vi "CAN路测试.vi"(5 "滤波方式":u8(ring) items=["Dual Filter", "Single Filter"], 6 "E-U_baud":u32(ring)=393223 items=["0x060003--1000Kbps"=393219, "0x060004--800Kbps"=393220, "0x060007--500Kbps"=393223, "0x1C0008--250Kbps"=1835016, "0x1C0011--125Kbps"=1835025, "0x160023--100Kbps"=1441827, "0x1C002C--50Kbps"=1835052, "0x1600B3--20Kbps"=1441971, "0x1C00E0--10Kbps"=1835232, "0x1C01C1--5Kbps"=1835457], 7 "工作方式":u8(ring) items=["Normal", "Listen Only"], 8 "波特率":T1(ring)=enum."500Kbps", 9 "CAN端口":u16(ring) items=["0", "1"], 10 "设备索引号":u16(ring) items=["0", "1", "2", "3", "4", "5", "6", "7", "8", "9", "10", "11", "12", "13", "14", "15", ""], 11 "CAN卡类型":u32(ring)=4 items=["PCI5121"=1, "PCI9810"=2, "USBCAN1"=3, "USBCAN2"=4, "PCI9820"=5, "PCI5110"=7, "CANLite(mini)"=8, "ISA9620"=9, "ISA5420"=10, "PC104CAN"=11, "DNP9810"=13, "PCI9840B"=14, "PC104C2"=15, "PCI9820I"=16, "pec9920"=18, "USBCAN_E_U"=20, "USBCAN_2E_U"=21]) -> ()   [LabVIEW 2013]
uses:
  data/kerneldlls/usbcan.dll
panel:
  in  "数值 4":i32
  in  "数值 3":i32
  out "错误输出":errorcluster
  in  "数值 2":i32
  in  "数值":i32
  in  "退出":bool
  out "整车CAN测试结果":bool
  out "充电CAN测试结果":bool
  out "结果":i32(listbox)=-1
  in  "充电CAN测试":bool
  in  "整车CAN测试":bool
  out "状态":string
  in  "启动CAN 2":bool caption="启动CAN"
  out "状态 2":bool
  out "CAN初始化成功":bool
  in  "启动CAN":bool
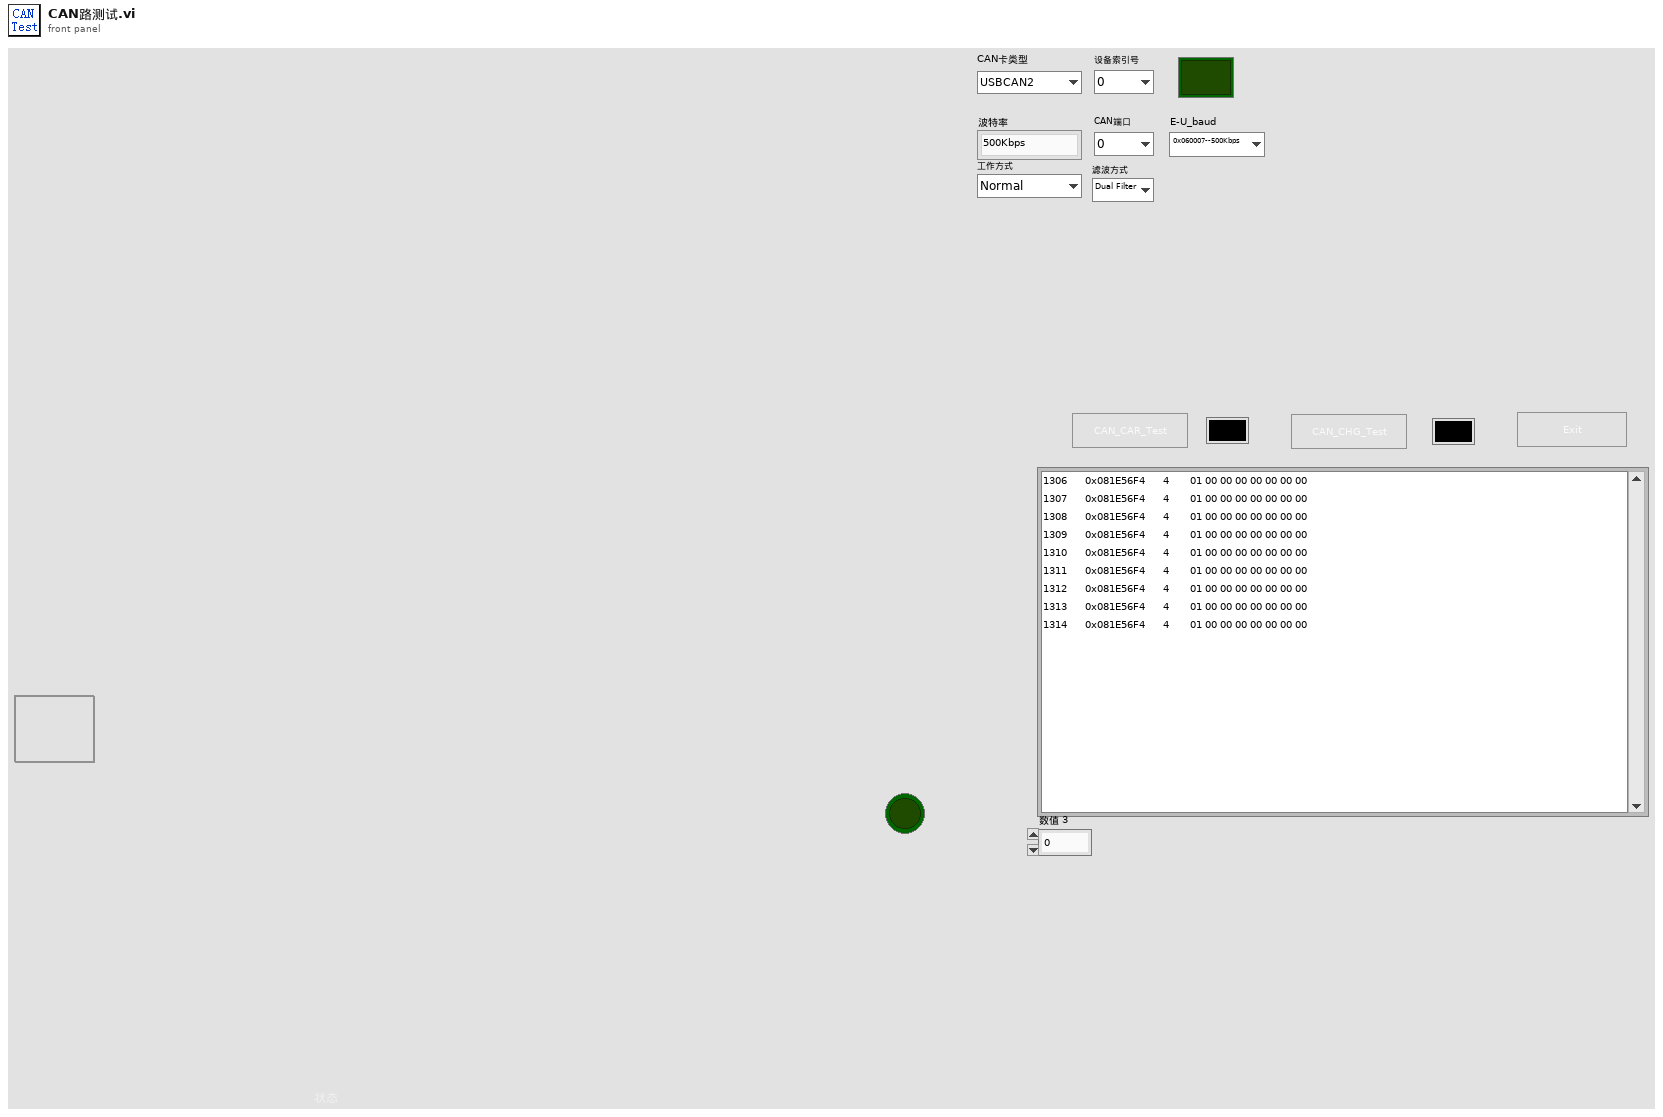
[diagram p1: front panel]
types:
  T1 = enum16{"5Kbps", "10Kbps", "20Kbps", "40Kbps", "50Kbps", "80Kbps", "100Kbps", "125Kbps", "200Kbps", "250Kbps", "400Kbps", "500Kbps", "666Kbps", "800Kbps", "1000Kbps"}
  T2 = cluster{"打开CAN":bool, "初始化CAN":bool, "开始CAN":bool, "重启":bool, "关闭CAN":bool}
  T3 = enum32{"Invalid", "Standard", "Closed", "Hidden", "Minimized", "Maximized"}
  T4 = cluster{"ID":u32, "TimeStamp":u32, "TimeFlag":u8, "SendType":u8, "RemoteFlag":u8, "ExternFlag":u8, "DataLen":u8, u8, u8, u8, u8, u8, u8, u8, u8, u8, u8, u8}[]
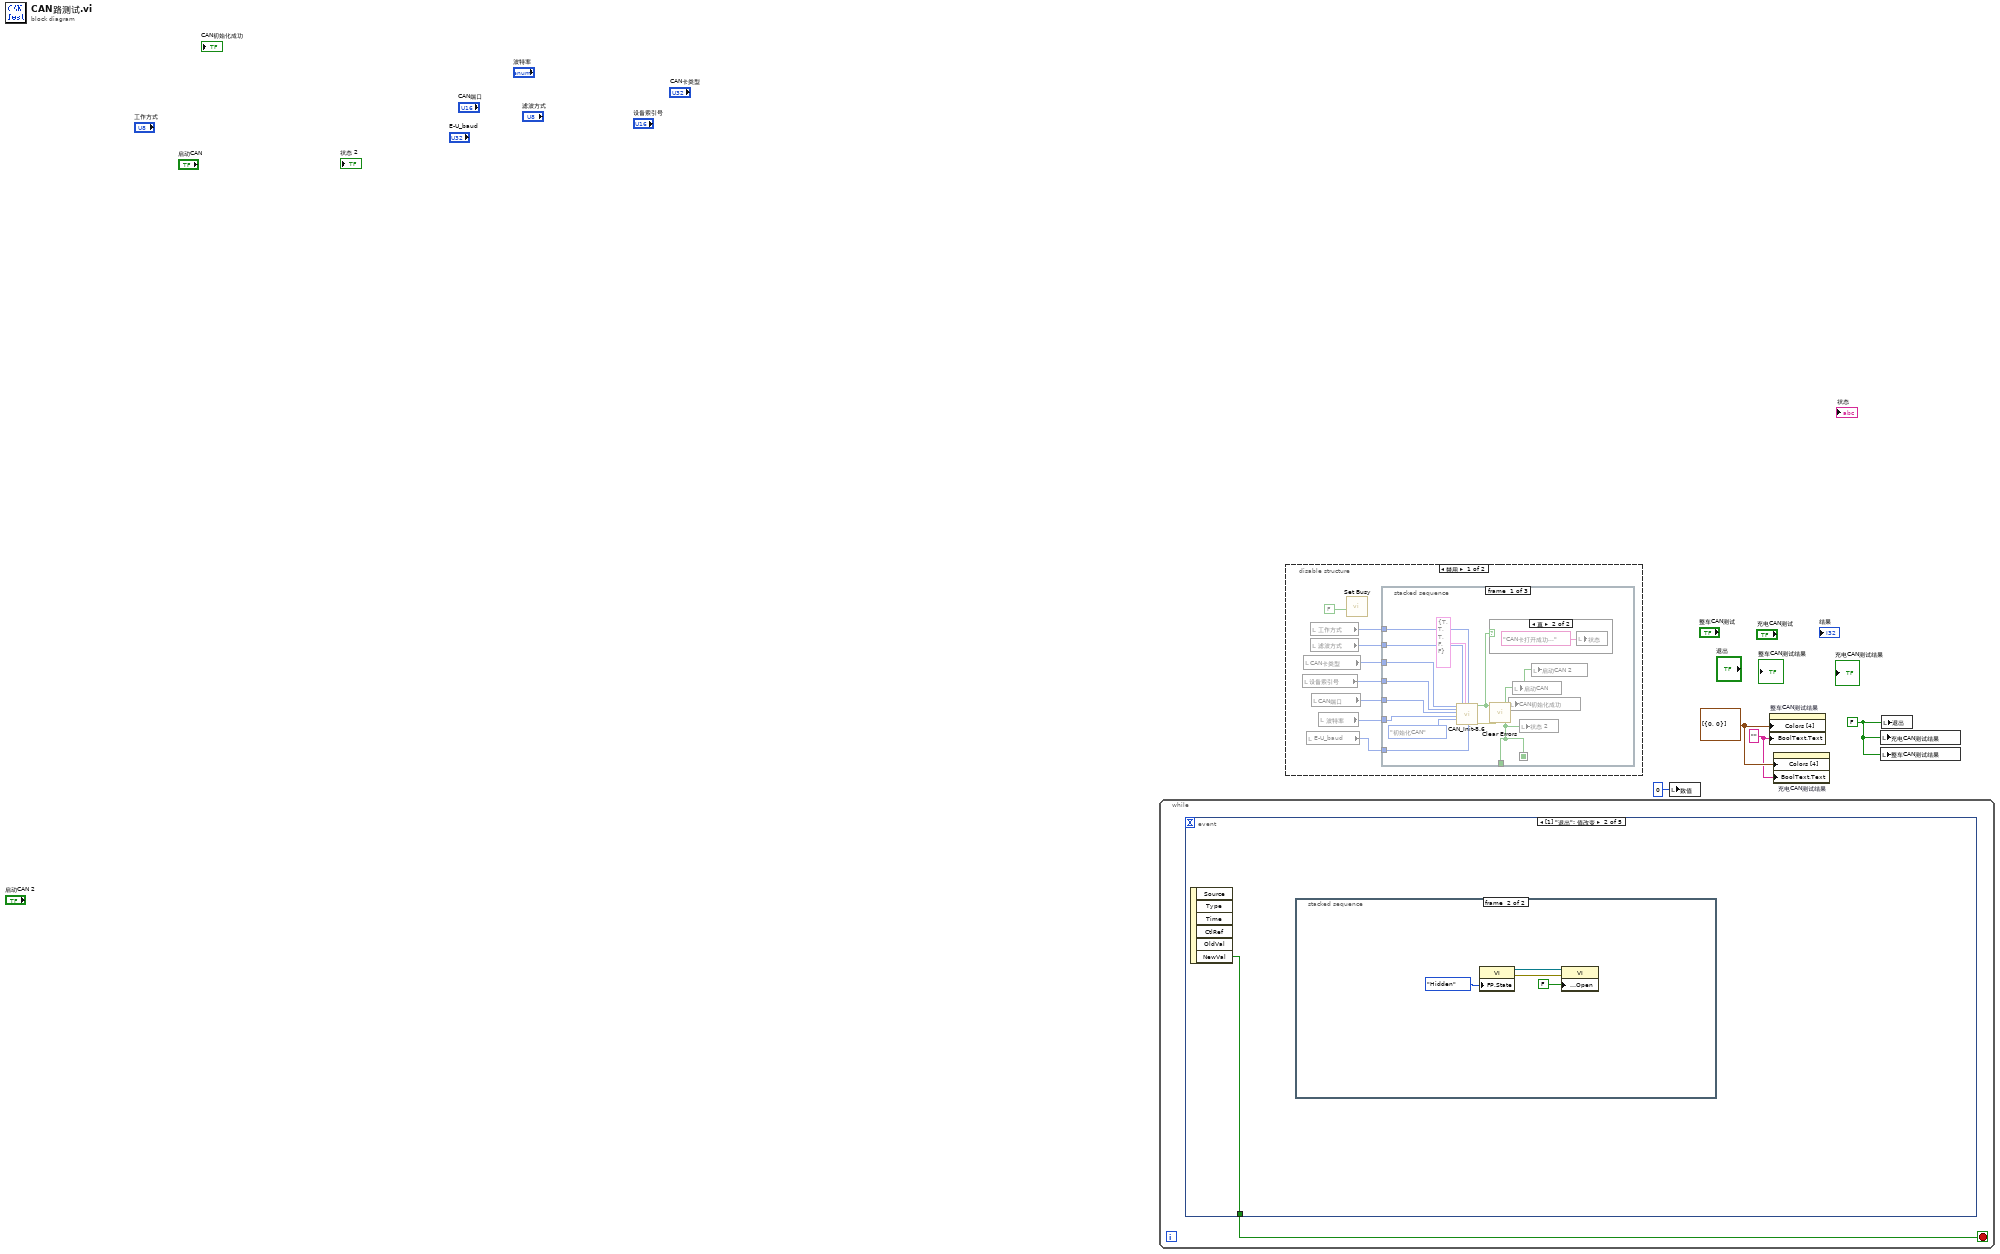
[diagram p0: block diagram]
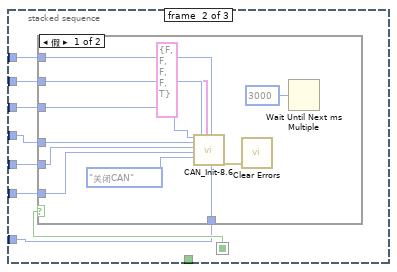
[diagram p3: hidden frame]
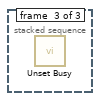
[diagram p5: hidden frame]
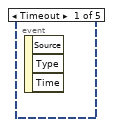
[diagram p7: hidden frame]
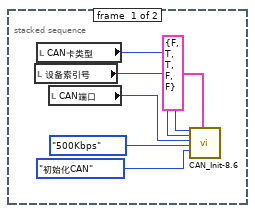
[diagram p8: hidden frame]
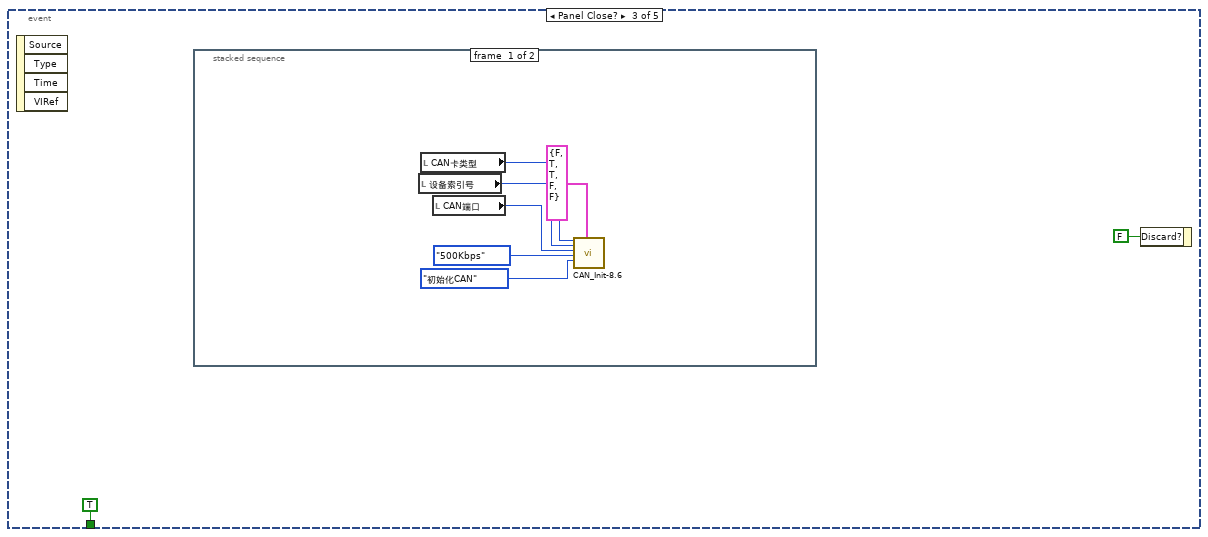
[diagram p9: hidden frame]
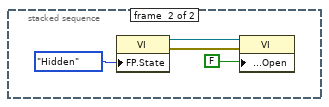
[diagram p10: hidden frame]
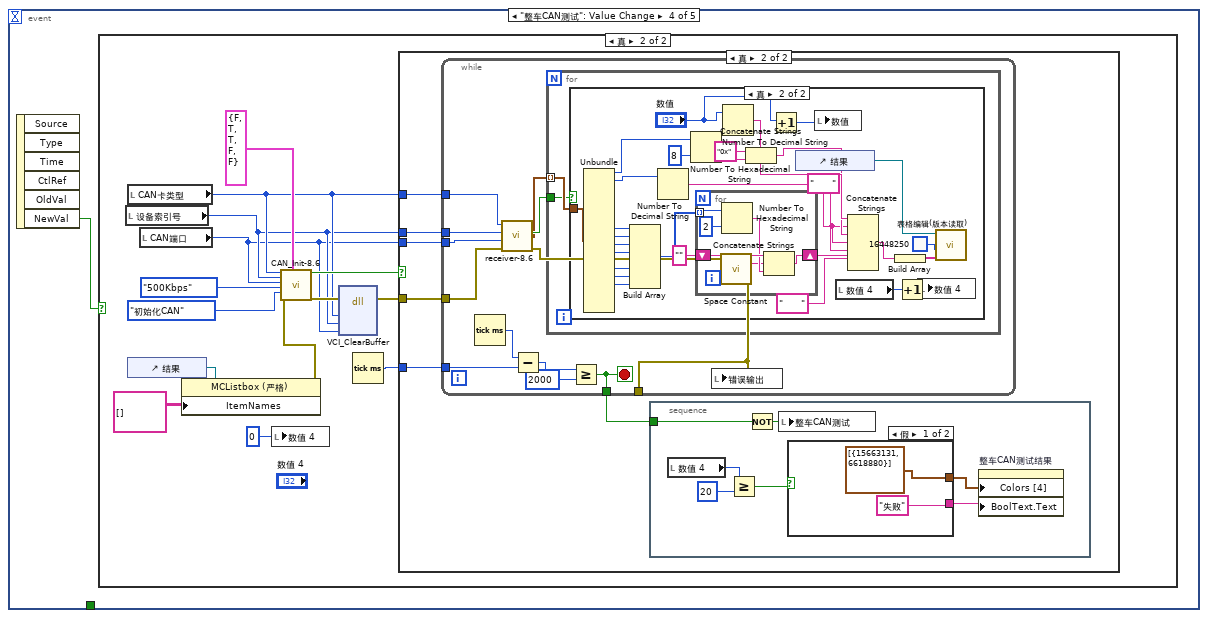
[diagram p11: hidden frame]
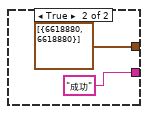
[diagram p14: hidden frame]
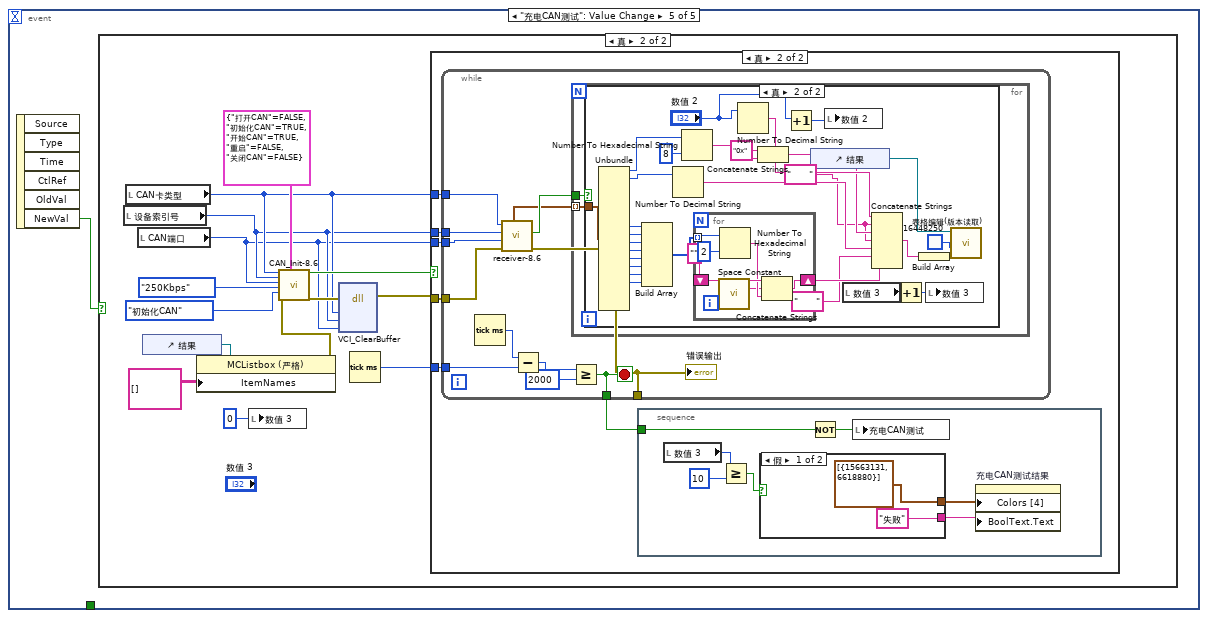
[diagram p16: hidden frame]
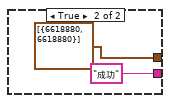
[diagram p19: hidden frame]
diagram:
  w1 = FALSE
  w2 = "" ("布尔文本.文本")
  w3 = cluster{u32, u32}[] [{0, 0}] ("颜色[4]")
  n1 = while {
    stop <- w5 stop-if-true
    n2 = event shown="[1] \"退出\": 值改变" {
      selector: _ -> [_ _ _ _ _]
      dyn-events: _ -> [_ _ _ _ _]
      timeout: _ -> [_ _ _ _ _]
      tunnel: [_ w6 TRUE ("NewVal") _ _] -> w5
      event Timeout {
        n3 = event-data() -> ()  [unwired: 1 in, 3 out]
      }
      event "退出": Value Change {
        n4 = event-data() -> ("NewVal"=w6:bool)  [unwired: 1 in, 5 out]
        n5 = stacked-sequence {
          frame #0 {
            n6 = local read "设备索引号"() -> (w9:u16)
            n7 = local read "CAN卡类型"() -> (w10:u32)
            n8 = local read "CAN端口"() -> (w8:u16)
            n9 = call "CAN_Init-8.6.vi"("CAN卡类型"=w10, "设备索引号"=w9, "CAN端口"=w8, "波特率"=T1."500Kbps", "操作类型"=enum16{"初始化CAN", "关闭CAN"}."初始化CAN", "簇"=T2 {"打开CAN"=FALSE, "初始化CAN"=TRUE, "开始CAN"=TRUE, "重启"=FALSE, "关闭CAN"=FALSE}) -> ()  [unwired: 8 in, 6 out]
          }
          frame #1 {
            n10 = property class="VI"("FP.State"=T3."Hidden" ("前面板窗口:状态")) -> (reference out=w15:refnum<vi>, error out=w16:errorcluster)  [unwired: 2 in]
            n11 = property class="VI"(reference=w15, error in=w16, "Front Panel.Open"=FALSE ("前面板窗口:打开")) -> ()  [unwired: 2 out]
          }
        }
      }
      event Panel Close? {
        n12 = event-data() -> ()  [unwired: 1 in, 4 out]
        n13 = stacked-sequence {
          frame #0 {
            n14 = local read "设备索引号"() -> (w21:u16)
            n15 = local read "CAN卡类型"() -> (w22:u32)
            n16 = local read "CAN端口"() -> (w20:u16)
            n17 = call "CAN_Init-8.6.vi"("CAN卡类型"=w22, "设备索引号"=w21, "CAN端口"=w20, "波特率"=T1."500Kbps", "操作类型"=enum16{"初始化CAN", "关闭CAN"}."初始化CAN", "簇"=T2 {"打开CAN"=FALSE, "初始化CAN"=TRUE, "开始CAN"=TRUE, "重启"=FALSE, "关闭CAN"=FALSE}) -> ()  [unwired: 8 in, 6 out]
          }
          frame #1 {
            n18 = property class="VI"("FP.State"=T3."Hidden" ("前面板窗口:状态")) -> (reference out=w27:refnum<vi>, error out=w28:errorcluster)  [unwired: 2 in]
            n19 = property class="VI"(reference=w27, error in=w28, "Front Panel.Open"=FALSE ("前面板窗口:打开")) -> ()  [unwired: 2 out]
          }
        }
        n20 = event-data("Discard?"=FALSE ("放弃？")) -> ()  [unwired: 1 in, 1 out]
      }
      event "整车CAN测试": Value Change {
        n21 = event-data() -> ("NewVal"=w29:bool)  [unwired: 1 in, 5 out]
        n22 = case shown="真" w29 {
          frame False {
          }
          frame True {
            n23 = local read "设备索引号"() -> (w32:u16)
            n24 = local read "CAN卡类型"() -> (w33:u32)
            n25 = control-ref of="结果"() -> (w38:refnum<vi>)
            n26 = local read "CAN端口"() -> (w31:u16)
            n27 = property class="MCListbox (严格)"(reference=w38, "ItemNames"=string[][] [] ("项名")) -> (error out=w36:errorcluster)  [unwired: 1 in, 1 out]
            n28 = local write "数值 4"(0 ("数值 4")) -> ()
            n29 = call "CAN_Init-8.6.vi"("CAN卡类型"=w33, "设备索引号"=w32, "CAN端口"=w31, "波特率"=T1."500Kbps", "操作类型"=enum16{"初始化CAN", "关闭CAN"}."初始化CAN", "error in (no error)"=w36, "簇"=T2 {"打开CAN"=FALSE, "初始化CAN"=TRUE, "开始CAN"=TRUE, "重启"=FALSE, "关闭CAN"=FALSE}) -> ("CAN 操作结果"=w40:bool, "error out"=w35:errorcluster)  [unwired: 7 in, 4 out]
            n30 = dll-call lib="PTH1aabs FBluewave New Energy\t上位机BMS_Monitor - 91版 新源data\nkerneldlls\nusbcan.dll" fn="VCI_ClearBuffer"(error in=w35, "DeviceType"=w33, "DeviceInd"=w32, "CANInd"=w31) -> (error out=w34:errorcluster)  [unwired: 3 in, 4 out]
            n31 = Tick Count (ms)() -> (millisecond timer value=w39:u32)
            n32 = case shown="真" w40 {
              tunnel: w33 -> [_ w46]
              tunnel: w32 -> [_ w45]
              tunnel: w31 -> [_ w44]
              tunnel: w39 -> [_ w49]
              tunnel: w34 -> [_ w47]
              frame False {
              }
              frame True {
                n33 = while {
                  tunnel: w46 -> [w72]
                  tunnel: w45 -> [w71]
                  tunnel: w44 -> [w70]
                  tunnel: w49 -> [w68]
                  tunnel: [w64] -> w48
                  tunnel: w47 -> [w63]
                  tunnel: [w62] -> _
                  stop <- w64 stop-if-true
                  n34 = Tick Count (ms)() -> (millisecond timer value=w69:u32)
                  n35 = call "receiver-8.6.vi"("错误输入（无错误）"=w63, "CAN端口"=w70, "设备索引号"=w71, "CAN卡类型"=w72) -> ("错误输出"=w62:errorcluster, "接收成功"=w65:bool, "VCI_CAN_OBJ_RN"=w61:T4)  [unwired: 3 out]
                  n36 = Subtract(x=w69, y=w68) -> (x-y=w67:u32)
                  n37 = for {
                    tunnel: w61 -> [w74] mode=indexing
                    tunnel: w65 -> [w73]
                    n38 = case shown="真" w73 {
                      tunnel: w74 -> [_ w104]
                      frame False {
                      }
                      frame True {
                        w85 = "      "
                        n39 = Unbundle(w104) -> ("ID"=w97:u32, "TimeStamp"=w96:u32, w82:u8, w81:u8, w80:u8, w79:u8, w78:u8, w77:u8, w76:u8, w75:u8)  [unwired: 8 out]
                        n40 = Build Array(w82, w81, w80, w79, w78, w77, w76, w75) -> (w103:u8[])
                        n41 = Number To Decimal String(number=w96) -> (decimal integer string=w95:string)  [unwired: 1 in]
                        n42 = Number To Hexadecimal String(1:i16 8 ("宽度(-)"), 2:w97) -> (0:w88:string)
                        n43 = for {
                          tunnel: w103 -> [w110] mode=indexing
                          shift-right: [w107] -> w94
                          shift-left: "" -> [w108]
                          n44 = call <vilib>:"Space Constant.vi"() -> ("String"=w105:string)
                          n45 = Number To Hexadecimal String(1:i16 2 ("宽度(-)"), 2:w110) -> (0:w106:string)
                          n46 = Concatenate Strings(w108, w105, w106) -> (w107:string)
                        }
                        n47 = Number To Decimal String(number="数值") -> (decimal integer string=w91:string)  [unwired: 1 in]
                        n48 = Concatenate Strings("0x" ("字符串"), w88) -> (w87:string)
                        n49 = Increment(x="数值") -> (x+1=w89:i32)
                        n50 = control-ref of="结果"() -> (w101:refnum<vi>)
                        n51 = local write "数值"(w89) -> ()
                        n52 = local read "数值 4"() -> (w84:i32)
                        n53 = Concatenate Strings(w91, w85, w87, w85, w95, "      ", w94) -> (w92:string)
                        n54 = Build Array(w92) -> (w100:string[])
                        n55 = Increment(x=w84) -> (x+1=w83:i32)
                        n56 = local write "数值 4"(w83) -> ()
                        n57 = call "表格编辑(版本读取).vi"("新元素/子数组"=w100, "活动单元格:单元格背景色"=u32 16448250, "MCListbox引用句柄"=w101) -> ()  [unwired: 9 in]
                      }
                    }
                  }
                  n58 = Greater Or Equal?(x=w67, y=u32 2000) -> (x >= y?=w64:bool)
                  n59 = local write "错误输出"(w62) -> ()
                }
                n60 = stacked-sequence {
                  tunnel: w48 -> [w56]
                  frame #0 {
                    n61 = local read "数值 4"() -> (w52:i32)
                    n62 = Greater Or Equal?(x=w52, y=20) -> (x >= y?=w50:bool)
                    n63 = Not(x=w56) -> (.not. x?=w55:bool)
                    n64 = local write "整车CAN测试"(w55) -> ()
                    n65 = case shown="假" w50 {
                      tunnel: [cluster{u32, u32}[] [{15663131, 6618880}] ("颜色[4]") cluster{u32, u32}[] [{6618880, 6618880}] ("颜色[4]")] -> w54
                      tunnel: ["失败" "成功"] -> w53
                      frame False {
                      }
                      frame True {
                      }
                    }
                    n66 = property on="整车CAN测试结果" class="Bool (严格)"("Colors [4]"=w54, "BoolText.Text"=w53) -> ()  [unwired: 2 in, 2 out]
                  }
                }
              }
            }
          }
        }
      }
      event "充电CAN测试": Value Change {
        n67 = event-data() -> ("NewVal"=w111:bool)  [unwired: 1 in, 5 out]
        n68 = case shown="真" w111 {
          frame False {
          }
          frame True {
            n69 = local read "设备索引号"() -> (w114:u16)
            n70 = local read "CAN卡类型"() -> (w115:u32)
            n71 = local read "CAN端口"() -> (w113:u16)
            n72 = control-ref of="结果"() -> (w120:refnum<vi>)
            n73 = property class="MCListbox (严格)"(reference=w120, "ItemNames"=string[][] [] ("项名")) -> (error out=w118:errorcluster)  [unwired: 1 in, 1 out]
            n74 = local write "数值 3"(0 ("数值 3")) -> ()
            n75 = call "CAN_Init-8.6.vi"("CAN卡类型"=w115, "设备索引号"=w114, "CAN端口"=w113, "波特率"=T1."250Kbps", "操作类型"=enum16{"初始化CAN", "关闭CAN"}."初始化CAN", "error in (no error)"=w118, "簇"=T2 {"打开CAN"=FALSE, "初始化CAN"=TRUE, "开始CAN"=TRUE, "重启"=FALSE, "关闭CAN"=FALSE}) -> ("CAN 操作结果"=w122:bool, "error out"=w117:errorcluster)  [unwired: 7 in, 4 out]
            n76 = dll-call lib="PTH1aabs FBluewave New Energy\t上位机BMS_Monitor - 91版 新源data\nkerneldlls\nusbcan.dll" fn="VCI_ClearBuffer"(error in=w117, "DeviceType"=w115, "DeviceInd"=w114, "CANInd"=w113) -> (error out=w116:errorcluster)  [unwired: 3 in, 4 out]
            n77 = Tick Count (ms)() -> (millisecond timer value=w121:u32)
            n78 = case shown="真" w122 {
              tunnel: w115 -> [_ w128]
              tunnel: w114 -> [_ w127]
              tunnel: w113 -> [_ w126]
              tunnel: w121 -> [_ w131]
              tunnel: w116 -> [_ w129]
              frame False {
              }
              frame True {
                n79 = while {
                  tunnel: w128 -> [w154]
                  tunnel: w127 -> [w153]
                  tunnel: w126 -> [w152]
                  tunnel: w131 -> [w150]
                  tunnel: [w146] -> w130
                  tunnel: w129 -> [w145]
                  tunnel: [w144] -> _
                  stop <- w146 stop-if-true
                  n80 = Tick Count (ms)() -> (millisecond timer value=w151:u32)
                  n81 = call "receiver-8.6.vi"("错误输入（无错误）"=w145, "CAN端口"=w152, "设备索引号"=w153, "CAN卡类型"=w154) -> ("错误输出"=w144:errorcluster, "接收成功"=w147:bool, "VCI_CAN_OBJ_RN"=w143:T4)  [unwired: 3 out]
                  "错误输出" <- w144
                  n82 = Subtract(x=w151, y=w150) -> (x-y=w149:u32)
                  n83 = Greater Or Equal?(x=w149, y=u32 2000) -> (x >= y?=w146:bool)
                  n84 = for {
                    tunnel: w143 -> [w156] mode=indexing
                    tunnel: w147 -> [w155]
                    n85 = case shown="真" w155 {
                      tunnel: w156 -> [_ w186]
                      frame False {
                      }
                      frame True {
                        w167 = "      "
                        n86 = Unbundle(w186) -> ("ID"=w179:u32, "TimeStamp"=w178:u32, w164:u8, w163:u8, w162:u8, w161:u8, w160:u8, w159:u8, w158:u8, w157:u8)  [unwired: 8 out]
                        n87 = Build Array(w164, w163, w162, w161, w160, w159, w158, w157) -> (w185:u8[])
                        n88 = Number To Decimal String(number=w178) -> (decimal integer string=w176:string)  [unwired: 1 in]
                        n89 = Number To Hexadecimal String(1:i16 8 ("宽度(-)"), 2:w179) -> (0:w177:string)
                        n90 = for {
                          tunnel: w185 -> [w192] mode=indexing
                          shift-right: [w189] -> w175
                          shift-left: "" -> [w190]
                          n91 = call <vilib>:"Space Constant.vi"() -> ("String"=w187:string)
                          n92 = Number To Hexadecimal String(1:i16 2 ("宽度(-)"), 2:w192) -> (0:w188:string)
                          n93 = Concatenate Strings(w190, w187, w188) -> (w189:string)
                        }
                        n94 = Number To Decimal String(number="数值 2") -> (decimal integer string=w172:string)  [unwired: 1 in]
                        n95 = Concatenate Strings("0x" ("字符串"), w177) -> (w169:string)
                        n96 = Increment(x="数值 2") -> (x+1=w170:i32)
                        n97 = control-ref of="结果"() -> (w183:refnum<vi>)
                        n98 = local write "数值 2"(w170) -> ()
                        n99 = local read "数值 3"() -> (w166:i32)
                        n100 = Concatenate Strings(w172, w167, w169, w167, w176, "      ", w175) -> (w173:string)
                        n101 = Increment(x=w166) -> (x+1=w165:i32)
                        n102 = Build Array(w173) -> (w182:string[])
                        n103 = local write "数值 3"(w165) -> ()
                        n104 = call "表格编辑(版本读取).vi"("新元素/子数组"=w182, "活动单元格:单元格背景色"=u32 16448250, "MCListbox引用句柄"=w183) -> ()  [unwired: 9 in]
                      }
                    }
                  }
                }
                n105 = stacked-sequence {
                  tunnel: w130 -> [w138]
                  frame #0 {
                    n106 = local read "数值 3"() -> (w136:i32)
                    n107 = Greater Or Equal?(x=w136, y=10) -> (x >= y?=w134:bool)
                    n108 = case shown="假" w134 {
                      tunnel: [cluster{u32, u32}[] [{15663131, 6618880}] ("颜色[4]") cluster{u32, u32}[] [{6618880, 6618880}] ("颜色[4]")] -> w133
                      tunnel: ["失败" "成功"] -> w132
                      frame False {
                      }
                      frame True {
                      }
                    }
                    n109 = Not(x=w138) -> (.not. x?=w137:bool)
                    n110 = local write "充电CAN测试"(w137) -> ()
                    n111 = property on="充电CAN测试结果" class="Bool (严格)"("Colors [4]"=w133, "BoolText.Text"=w132) -> ()  [unwired: 2 in, 2 out]
                  }
                }
              }
            }
          }
        }
      }
    }
  }
  n112 = disable-structure shown="禁用" {
    frame Disabled {
      n113 = local read "设备索引号"() -> (w197:u16)
      n114 = local read "CAN卡类型"() -> (w198:u32)
      n115 = local read "E-U_baud"() -> (w194:u32)
      n116 = local read "工作方式"() -> (w200:u8)
      n117 = local read "滤波方式"() -> (w199:u8)
      n118 = local read "CAN端口"() -> (w196:u16)
      n119 = local read "波特率"() -> (w195:T1)
      n120 = call <vilib>:"Set Busy.vi"("disable click? (T)"=FALSE) -> ()  [unwired: 3 in, 8 out]
      n121 = stacked-sequence {
        seq-local: [w202 _ _] -> [_ w219 _]
        tunnel: [w202 _ _] -> _
        tunnel: w200 -> [w209 w220 _]
        tunnel: w199 -> [w208 w218 _]
        tunnel: w198 -> [w207 w217 _]
        tunnel: w197 -> [w206 w216 _]
        tunnel: w196 -> [w205 w215 _]
        tunnel: w195 -> [w204 w214 _]
        tunnel: w194 -> [w203 w213 _]
        frame #0 {
          n122 = call "CAN_Init-8.6.vi"("CAN卡类型"=w207, "设备索引号"=w206, "CAN端口"=w205, "波特率"=w204, "操作类型"=enum16{"初始化CAN", "关闭CAN"}."初始化CAN", "滤波方式"=w208, "簇"=T2 {"打开CAN"=TRUE, "初始化CAN"=TRUE, "开始CAN"=TRUE, "重启"=FALSE, "关闭CAN"=FALSE}, "工作方式"=w209, "E-U_baud"=w203) -> ("CAN 操作结果"=w202:bool, "error out"=w201:errorcluster)  [unwired: 5 in, 4 out]
          n123 = case shown="真" w202 {
            frame False {
            }
            frame True {
              n124 = local write "状态"("CAN卡打开成功..." ("状态")) -> ()
            }
          }
          n125 = call <vilib>:"Clear Errors.vi"("error in (no error)"=w201) -> ()  [unwired: 7 out]
          n126 = local write "CAN初始化成功"(w202) -> ()
          n127 = local write "启动CAN"(w202) -> ()
          n128 = local write "状态 2"(w202) -> ()
          n129 = local write "启动CAN 2"(w202) -> ()
        }
        frame #1 {
          n130 = case shown="假" w219 {
            tunnel: w220 -> [w231 _]
            tunnel: w218 -> [w230 _]
            tunnel: w217 -> [w229 _]
            tunnel: w216 -> [w228 _]
            tunnel: w215 -> [w227 _]
            tunnel: w214 -> [w226 _]
            tunnel: w213 -> [w225 _]
            frame False {
              n131 = call "CAN_Init-8.6.vi"("CAN卡类型"=w229, "设备索引号"=w228, "CAN端口"=w227, "波特率"=w226, "操作类型"=enum16{"初始化CAN", "关闭CAN"}."关闭CAN", "滤波方式"=w230, "簇"=T2 {"打开CAN"=FALSE, "初始化CAN"=FALSE, "开始CAN"=FALSE, "重启"=FALSE, "关闭CAN"=TRUE}, "工作方式"=w231, "E-U_baud"=w225) -> ("error out"=w221:errorcluster)  [unwired: 5 in, 5 out]
              n132 = call <vilib>:"Clear Errors.vi"("error in (no error)"=w221) -> ()  [unwired: 7 out]
              n133 = Wait Until Next ms Multiple(millisecond multiple=u32 3000 ("毫秒倍数")) -> ()  [unwired: 1 out]
            }
            frame True {
            }
          }
        }
        frame #2 {
          n134 = call <vilib>:"Unset Busy.vi"() -> ()  [unwired: 2 in, 10 out]
        }
      }
    }
    frame Enabled {
    }
  }
  n135 = local write "数值"(0 ("数值")) -> ()
  n136 = property on="整车CAN测试结果" class="Bool (严格)"("Colors [4]"=w3, "BoolText.Text"=w2) -> ()  [unwired: 2 in, 2 out]
  n137 = property on="充电CAN测试结果" class="Bool (严格)"("Colors [4]"=w3, "BoolText.Text"=w2) -> ()  [unwired: 2 in, 2 out]
  n138 = local write "充电CAN测试结果"(w1) -> ()
  n139 = local write "整车CAN测试结果"(w1) -> ()
  n140 = local write "退出"(w1) -> ()
